vi "databasePath.vi"() -> ()   [LabVIEW 2011]
panel:
  in  "database backup PATH":string="C:\\HVAC\\database_backup"
  in  "database PATH":string="C:\\HVAC\\database\\mydatabase.sqlite"
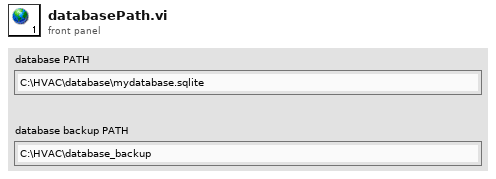
[diagram p1: front panel]
diagram:
